vi "Get Path Regex.vi"(8 "error in (no error)":errorcluster, 11 "Approval in":refnum<class "Approval.lvclass">) -> (0 "error out":errorcluster, 2 "Path Regex":string, 3 "Approval out":refnum<class "Approval.lvclass">)   [LabVIEW 2020, in "Summer of LabVIEW.lvlib" / "Approval.lvclass"]
uses:
  Approval.lvclass
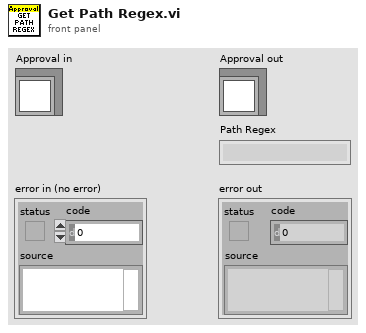
[diagram p1: front panel]
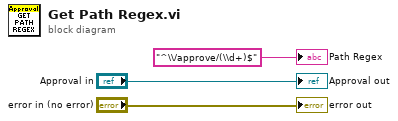
[diagram p0: block diagram]
diagram:
  "error out" <- "error in (no error)"
  "Approval out" <- "Approval in"
  "Path Regex" <- "^\\/approve/(\\d+)$" ("Path Regex")
